vi "Read Connection List.vi"(8 "error in (no error)":errorcluster, 11 "Switch Connect Message in":refnum<class "Switch Connect Message.lvclass">) -> (0 "error out":errorcluster, 2 "Connection List":string, 3 "Switch Connect Message out":refnum<class "Switch Connect Message.lvclass">)   [LabVIEW 2027, in "Messaging.lvlib" / "Switch Connect Message.lvclass"]
uses:
  Switch Connect Message.lvclass
  Switch Connect Message.lvclass/Switch Connect Message.ctl
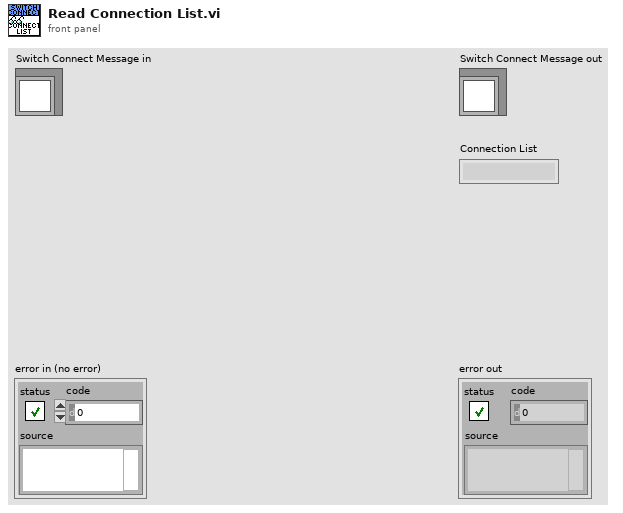
[diagram p1: front panel]
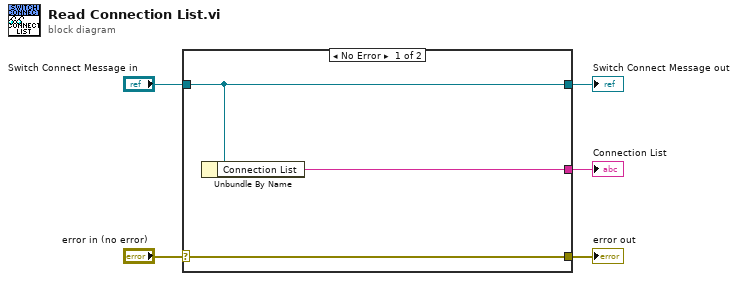
[diagram p0: block diagram]
diagram:
  n1 = case shown="No Error" "error in (no error)" {
    selector: "error in (no error)" -> [w8 w9]
    tunnel: [w8 w9] -> w4
    tunnel: [w7 w10] -> w2
    tunnel: "Switch Connect Message in" -> [w7 w10]
    tunnel: [w6 _] -> w1
    frame No Error {
      n2 = Unbundle By Name(w7) -> ("Connection List"=w6:string)
    }
    frame Error {
    }
  }
  "error out" <- w4
  "Switch Connect Message out" <- w2
  "Connection List" <- w1
